vi "Dispense FN - OFF - Measure Slope -2 (SubVI).vi"(0 "Settings":T1={"ON Settings"={"Enable Dynamic Setpoint?"=TRUE, "Enable Dynamic Dispense Time?"=TRUE, "Enable Drain Rate Functions"=TRUE, "Dispense Sample Time (s)"=0.1, "Mass Average Samples"=20, "ON Timeout (sec)"=300.0, "1st Setpoint (% of Target)"=90.0, "2nd Setpoint (% of Target)"=95.0, "3rd Setpoint (% of Target)"=100.0, "Measure Dispense Delay (sec)"=10.0, "Minimum Spray Time (s)"=2.0, "Pump Reverse Time (s)"=10.0}, "OFF Settings"={"Drain Sample Time (s)"=0.1, "Drain Rate Ave Size"=100, "Drain Rate Limits (± g/sec)"=100.0, "Level Slope Range (± g/sec)"=0.05, "OFF Timeout (sec)"=300.0, "Near SP Slope Level (± g/sec)"=0.005, "Near Setpoint Threshold (%)"=99.0}, "Overshoot Settings"={"Time Limit (s)"=30.0, "Container MAX (g)"=1500.0, "Max FILL Slope (+/- g/sec)"=100.0, "% Overshot to Enable (>)"=3.0}, "FILL Timeout (s)"=300.0, "Full \nSettle Time (s)"=30.0, "Pre-Hydrate \nSpray Time (s)"=0.0, "Pre-Hydrate \nWait Time (s)"=10.0, "m Value "=1.0, "b Value"=0.0, "Enable Overshoot Adjust?"=FALSE} {"ON Settings"."Pump Reverse Time (s)" min=0.0 max=60.0; "OFF Settings"."Near SP Slope Level (± g/sec)" format="%.3g"; "OFF Settings"."Level Slope Range (± g/sec)" format="%.3g"}, 1 "Initialize":bool, 2 "Measured Mass (g)":dbl, 5 "Static Setpoint (g)":dbl, 7 "Sample?":bool, 9 "Max Drain Complete?":bool, 11 "Elapsed Time (s)":dbl) -> (14 "Level Signal":bool, 15 "Drain Time (s)":dbl, 16 "Drain Rate (g/sec)":dbl, 17 "Ave. Slope (g/sec)":dbl)   [LabVIEW 2011]
uses:
  <vilib>/ptbypt/NI_PtbyPt.lvlib
panel:
  out "Level Count":i32
  # "ONLY ADJUST\nBOLD VALUES!"
  # "Corrected Mass = SDC Mass * m + b"
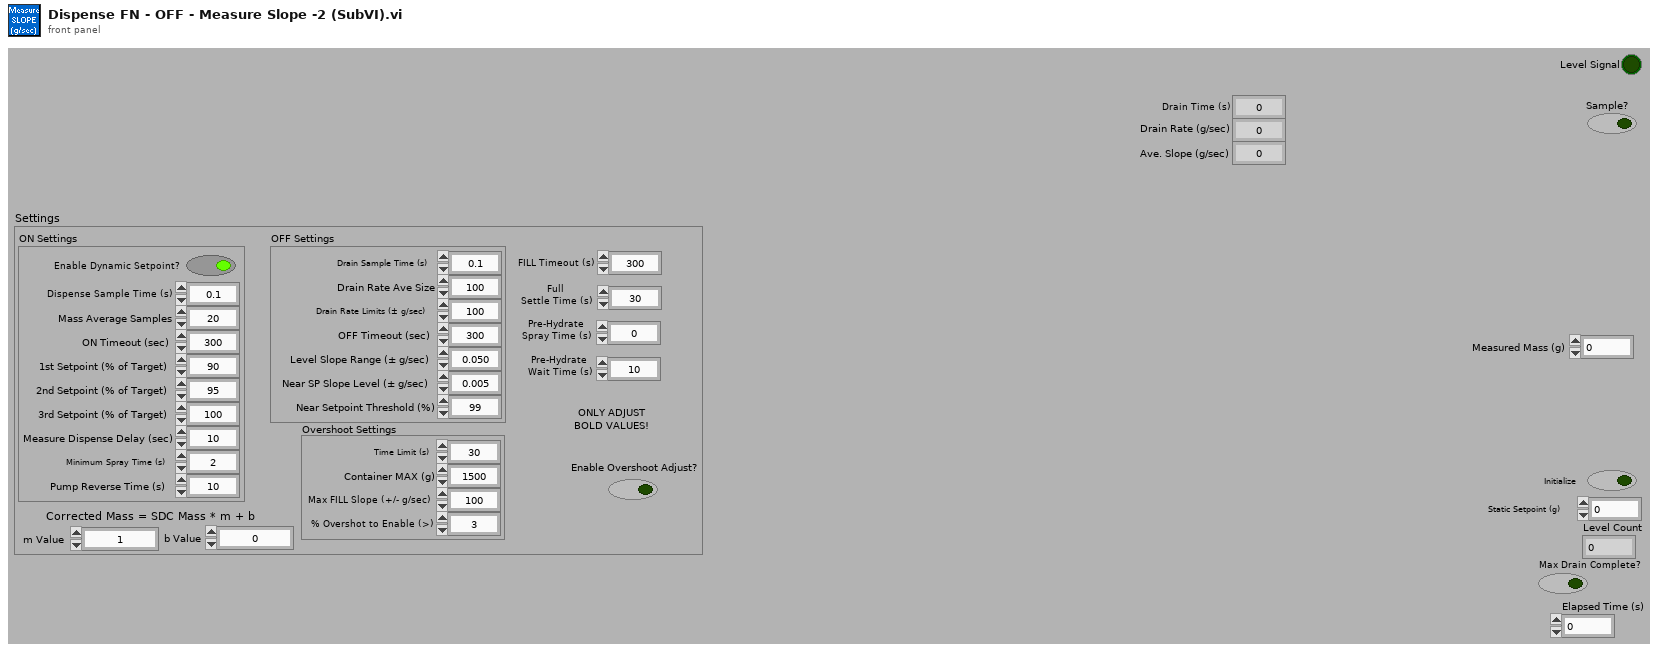
[diagram p1: front panel]
types:
  T1 = cluster{"ON Settings":cluster{"Enable Dynamic Setpoint?":bool, "Enable Dynamic Dispense Time?":bool, "Enable Drain Rate Functions":bool, "Dispense Sample Time (s)":dbl, "Mass Average Samples":i32, "ON Timeout (sec)":dbl, "1st Setpoint (% of Target)":dbl, "2nd Setpoint (% of Target)":dbl, "3rd Setpoint (% of Target)":dbl, "Measure Dispense Delay (sec)":dbl, "Minimum Spray Time (s)":dbl, "Pump Reverse Time (s)":dbl}, "OFF Settings":cluster{"Drain Sample Time (s)":dbl, "Drain Rate Ave Size":i32, "Drain Rate Limits (± g/sec)":dbl, "Level Slope Range (± g/sec)":dbl, "OFF Timeout (sec)":dbl, "Near SP Slope Level (± g/sec)":dbl, "Near Setpoint Threshold (%)":dbl}, "Overshoot Settings":cluster{"Time Limit (s)":dbl, "Container MAX (g)":dbl, "Max FILL Slope (+/- g/sec)":dbl, "% Overshot to Enable (>)":dbl}, "FILL Timeout (s)":dbl, "Full \nSettle Time (s)":dbl, "Pre-Hydrate \nSpray Time (s)":dbl, "Pre-Hydrate \nWait Time (s)":dbl, "m Value ":dbl, "b Value":dbl, "Enable Overshoot Adjust?":bool}
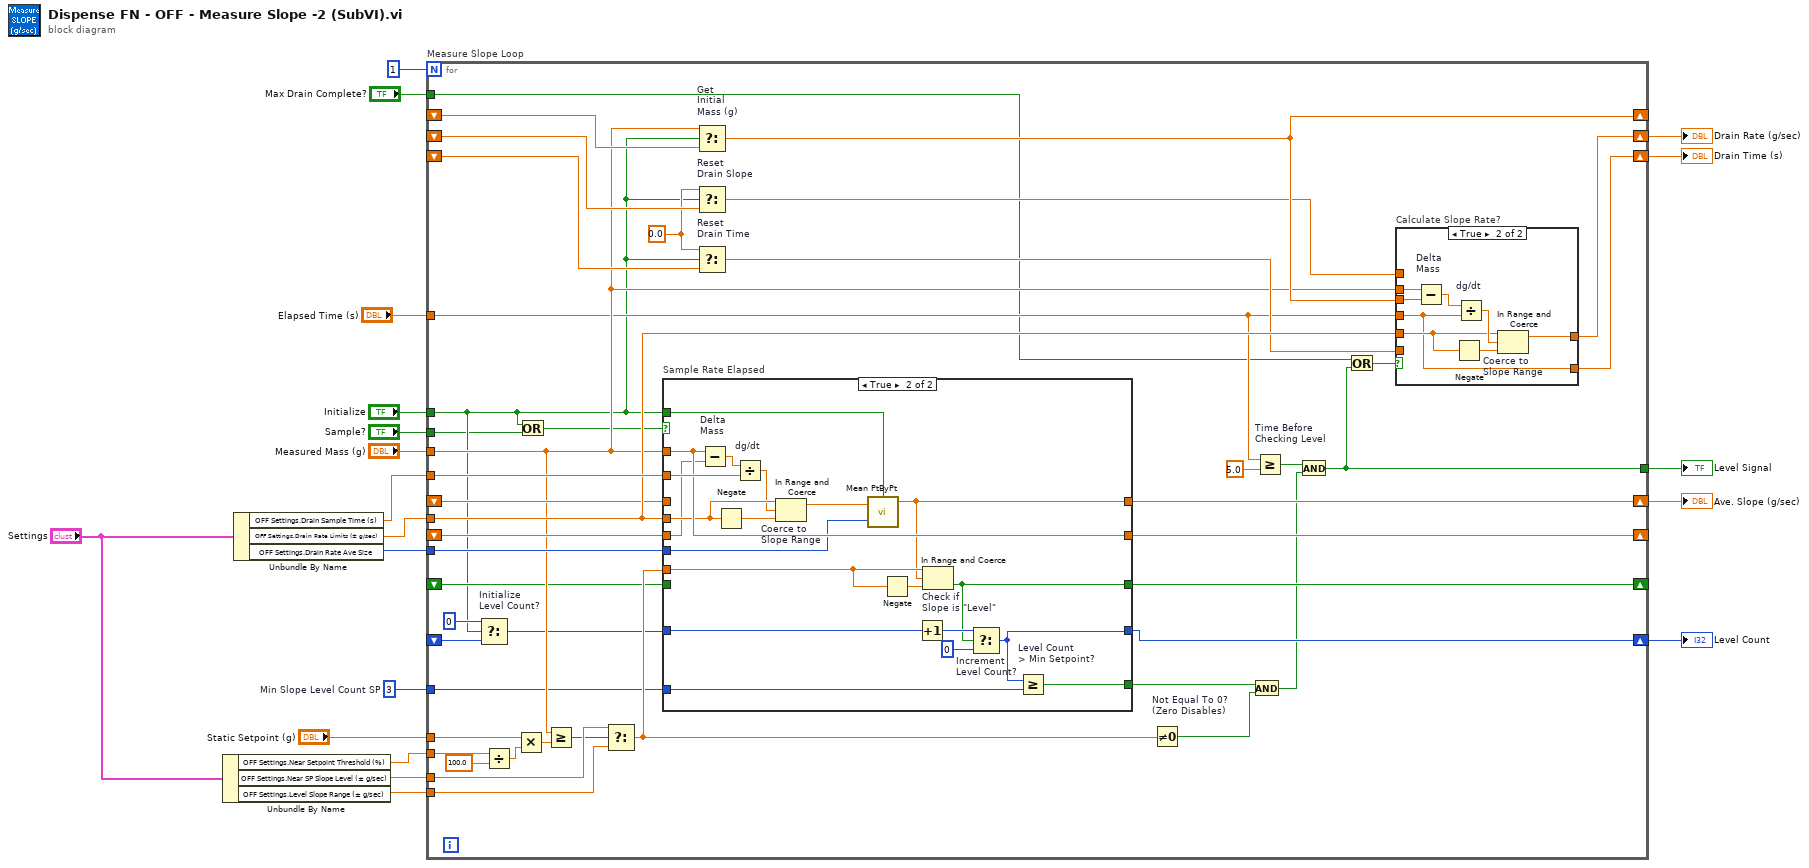
[diagram p0: block diagram]
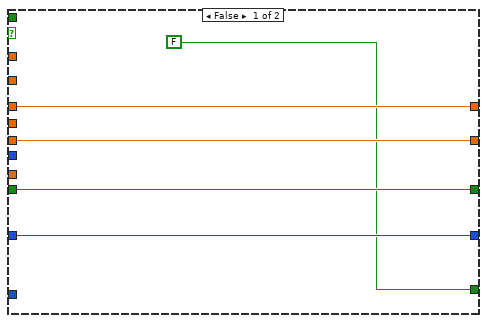
[diagram p3: hidden frame]
diagram:
  w7 = 3  # Min Slope Level Count SP
  n1 = Unbundle By Name("Settings") -> ("OFF Settings.Near Setpoint Threshold (%)"=w13:dbl, "OFF Settings.Near SP Slope Level (± g/sec)"=w12:dbl, "OFF Settings.Level Slope Range (± g/sec)"=w11:dbl)
  n2 = Unbundle By Name("Settings") -> ("OFF Settings.Drain Sample Time (s)"=w10:dbl, "OFF Settings.Drain Rate Limits (± g/sec)"=w9:dbl, "OFF Settings.Drain Rate Ave Size"=w8:i32)
  n3 = for "Measure Slope Loop" {
    N: 1 -> [_]
    tunnel: "Measured Mass (g)" -> [w42]
    shift-right: [w65] -> _
    shift-left: _ -> [w51]
    shift-right: [w52] -> w19
    shift-left: _ -> [w50]
    tunnel: w10 -> [w63]
    tunnel: "Initialize" -> [w23]
    tunnel: w9 -> [w60]
    tunnel: w12 -> [w41]
    tunnel: w8 -> [w64]
    shift-right: [w61] -> _
    shift-left: _ -> [w62]
    shift-right: [w59] -> w16
    shift-left: _ -> [w58]
    shift-right: [w56] -> w2
    shift-left: _ -> [w55]
    tunnel: [w27] -> w15
    tunnel: "Static Setpoint (g)" -> [w47]
    tunnel: w13 -> [w45]
    tunnel: w11 -> [w40]
    shift-right: [w38] -> w6
    shift-left: _ -> [w36]
    shift-right: [w34] -> _
    shift-left: _ -> [w33]
    tunnel: w7 -> [w32]
    tunnel: "Elapsed Time (s)" -> [w25]
    tunnel: "Sample?" -> [w21]
    tunnel: "Max Drain Complete?" -> [w24]
    w54 = 0.0 ("t")
    n4 = Select "Initialize\nLevel Count?"(t=0 ("f"), s=w23, f=w36) -> (s? t:f=w35:i32)
    n5 = Divide(x=w45, y=100.0) -> (x/y=w44:dbl)
    n6 = Multiply(x=w47, y=w44) -> (x*y=w43:dbl)
    n7 = Or(x=w23, y=w21) -> (x .or. y?=w22:bool)
    n8 = Greater Or Equal?(x=w42, y=w43) -> (x >= y?=w26:bool)
    n9 = Select(t=w41, s=w26, f=w40) -> (s? t:f=w39:dbl)
    n10 = case "Sample Rate Elapsed" shown="True" w22 {
      tunnel: w42 -> [_ w98]
      tunnel: [w80 w88] -> w52
      tunnel: [w79 w98] -> w65
      tunnel: w63 -> [_ w99]
      tunnel: w60 -> [_ w97]
      tunnel: w64 -> [_ w95]
      tunnel: w23 -> [_ w94]
      tunnel: w51 -> [w79 w93]
      tunnel: w50 -> [w80 _]
      tunnel: w39 -> [_ w89]
      tunnel: w35 -> [w78 w86]
      tunnel: [w78 w84] -> w38
      tunnel: [w77 w83] -> w34
      tunnel: [FALSE w82] -> w31
      tunnel: w33 -> [w77 _]
      tunnel: w32 -> [_ w81]
      frame False {
      }
      frame True {
        n11 = Subtract "Delta\nMass"(x=w98, y=w93) -> (x-y=w100:dbl)
        n12 = Negate(x=w97) -> (-x=w96:dbl)
        n13 = Divide "dg/dt"(x=w100, y=w99) -> (x/y=w91:dbl)
        n14 = In Range and Coerce "Coerce to\nSlope Range"(upper limit=w97, x=w91, lower limit=w96) -> (coerced(x)=w92:dbl)  [unwired: 1 out]
        n15 = call <vilib>:"Mean PtByPt.vi"("x"=w92, "sample length"=w95, "initialize"=w94) -> ("mean"=w88:dbl)  [unwired: 2 out]
        n16 = Negate(x=w89) -> (-x=w90:dbl)
        n17 = Increment(x=w86) -> (x+1=w87:i32)
        n18 = In Range and Coerce "Check if\nSlope is \"Level\""(upper limit=w89, x=w88, lower limit=w90) -> (In Range?=w83:bool)  [unwired: 1 out]
        n19 = Select "Increment\nLevel Count?"(t=w87, s=w83, f=0) -> (s? t:f=w84:i32)
        n20 = Greater Or Equal? "Level Count\n> Min Setpoint?"(x=w84, y=w81) -> (x >= y?=w82:bool)
      }
    }
    n21 = Select "Get\nInitial\nMass (g)"(t=w42, s=w23, f=w62) -> (s? t:f=w61:dbl)
    n22 = Select "Reset\nDrain Slope"(t=w54, s=w23, f=w58) -> (s? t:f=w57:dbl)
    n23 = Select "Reset\nDrain Time"(t=w54, s=w23, f=w55) -> (s? t:f=w53:dbl)
    n24 = Not Equal To 0? "Not Equal To 0?\n(Zero Disables)"(x=w39) -> (x != 0?=w30:bool)
    n25 = And(x=w31, y=w30) -> (x .and. y?=w28:bool)
    n26 = Greater Or Equal? "Time Before\nChecking Level"(x=w25, y=5.0) -> (x >= y?=w29:bool)
    n27 = And(x=w29, y=w28) -> (x .and. y?=w27:bool)
    n28 = Or(x=w24, y=w27) -> (x .or. y?=w48:bool)
    n29 = case "Calculate Slope Rate?" shown="True" w48 {
      tunnel: w42 -> [_ w73]
      tunnel: w61 -> [_ w69]
      tunnel: w25 -> [_ w68]
      tunnel: w60 -> [_ w71]
      tunnel: [w67 w70] -> w59
      tunnel: w57 -> [w67 _]
      tunnel: [w66 w68] -> w56
      tunnel: w53 -> [w66 _]
      frame False {
      }
      frame True {
        n30 = Subtract "Delta\nMass"(x=w73, y=w69) -> (x-y=w72:dbl)
        n31 = Negate(x=w71) -> (-x=w75:dbl)
        n32 = Divide "dg/dt"(x=w72, y=w68) -> (x/y=w74:dbl)
        n33 = In Range and Coerce "Coerce to\nSlope Range"(upper limit=w71, x=w74, lower limit=w75) -> (coerced(x)=w70:dbl)  [unwired: 1 out]
      }
    }
  }
  "Ave. Slope (g/sec)" <- w19
  "Level Signal" <- w15
  "Drain Rate (g/sec)" <- w16
  "Level Count" <- w6
  "Drain Time (s)" <- w2
